vi "Teleop_DriveFwd.vi"   [LabVIEW 2017]
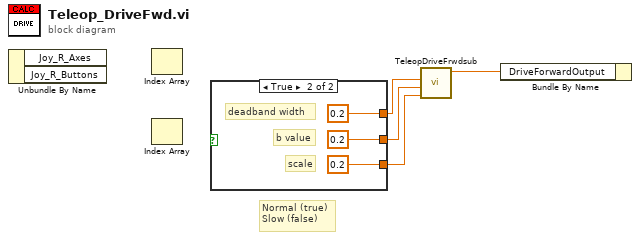
[diagram p0: block diagram]
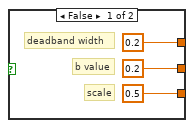
[diagram p2: hidden frame]
diagram:
  # "Normal (true)\nSlow (false)"
  n1 = Unbundle By Name() -> ()  [unwired: 1 in, 2 out]
  n2 = Index Array() -> ()  [unwired: 2 in, 1 out]
  n3 = Index Array() -> ()  [unwired: 2 in, 1 out]
  n4 = case shown="True" {
    selector: _ -> [_ _]
    tunnel: [0.5 ("a value") 0.2 ("a value")] -> w4
    tunnel: [0.2 ("b value") 0.2 ("dead band val")] -> w3
    tunnel: [0.2 ("dead band val") 0.2 ("b value")] -> w2
    frame False {
      # "scale"
      # "b value"
      # "deadband width"
    }
    frame True {
      # "scale"
      # "b value"
      # "deadband width"
    }
  }
  n5 = call "TeleopDriveFrwdsub.vi"("SCALE"=w4, "B VALUE"=w3, "Deadband X value"=w2) -> ("Drive Output"=w1:dbl)  [unwired: 8 in]
  n6 = Bundle By Name("DriveForwardOutput"=w1) -> ()  [unwired: 1 in, 1 out]
